vi "svpo_Average Array (real).vi"(6 "averages completed in":dbl, 7 "restart averaging":bool, 8 "exponential weight (10 %)":dbl=10.0 min=0.0 max=100.0 step=5.0, 9 "weighting mode":enum16{"Linear", "Exponential"}(ring), 10 "array":dbl[](array[numeric]) format="%.2p", 11 "previous average array":dbl[](array[numeric]) format="%.2p") -> (2 "averages completed out":dbl, 3 "average array":dbl[](array[numeric]) format="%.2p")   [LabVIEW 2017]
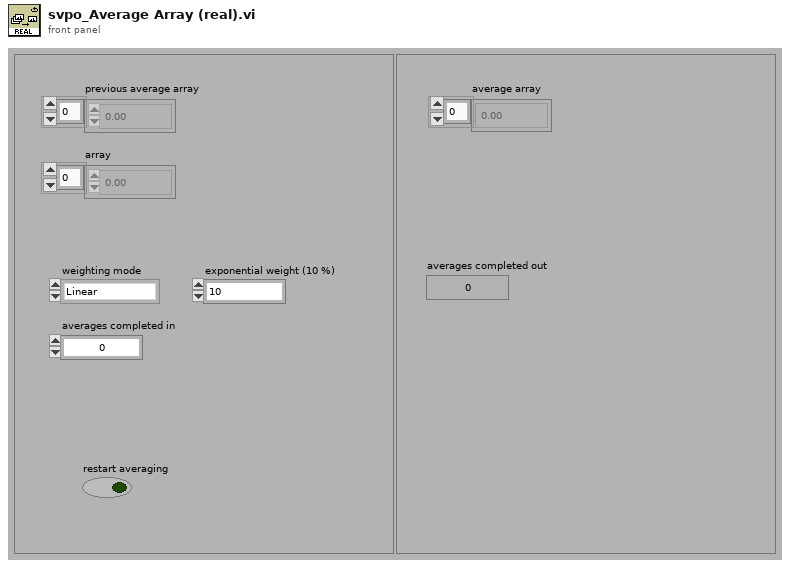
[diagram p1: front panel]
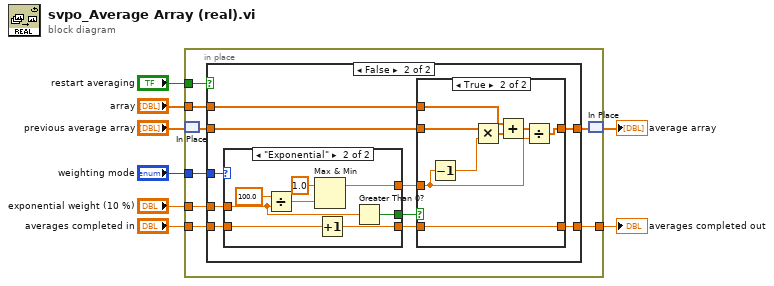
[diagram p0: block diagram]
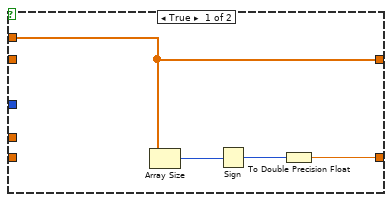
[diagram p2: hidden frame]
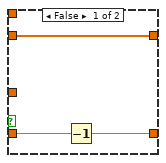
[diagram p3: hidden frame]
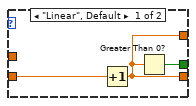
[diagram p4: hidden frame]
diagram:
  n1 = in-place {
    in-place-border: "weighting mode" -> [w16]
    in-place-border: "averages completed in" -> [w15]
    in-place-border: [w14] -> w6
    in-place-border: "array" -> [w13]
    in-place-border: "restart averaging" -> [w12]
    in-place-border: "exponential weight (10 %)" -> [w11]
    n2 = in-place-match #1("previous average array") -> (w10:dbl[])
    n3 = case shown="False" w12 {
      tunnel: [w19 w23] -> w14
      tunnel: w16 -> [_ w30]
      tunnel: w15 -> [_ w29]
      tunnel: w10 -> [_ w28]
      tunnel: w13 -> [w20 w27]
      tunnel: [w20 w26] -> w9
      tunnel: w11 -> [_ w25]
      frame True {
        n4 = Array Size(array=w20) -> (size(s)=w18:i32)
        n5 = Sign(1:w18) -> (0:w17:i32)
        n6 = To Double Precision Float(number=w17) -> (double precision float=w19:dbl)
      }
      frame False {
        n7 = case shown="\"Exponential\"" w30 {
          tunnel: w29 -> [w44 w51]
          tunnel: [w42 w52] -> w22
          tunnel: [w42 w48] -> w24
          tunnel: w25 -> [_ w46]
          tunnel: [w43 w45] -> w21
          frame "Linear", Default {
            n8 = Increment(x=w44) -> (x+1=w42:dbl)
            n9 = Greater Than 0?(x=w42) -> (x > 0?=w43:bool)
          }
          frame "Exponential" {
            n10 = Divide(x=100.0, y=w46) -> (x/y=w49:dbl)
            n11 = Max & Min(x=1.0 ("lower limit"), y=w49) -> (max(x,y)=w48:dbl)  [unwired: 1 out]
            n12 = Increment(x=w51) -> (x+1=w52:dbl)
            n13 = Greater Than 0?(x=w46) -> (x > 0?=w45:bool)
          }
        }
        n14 = case shown="True" w21 {
          tunnel: w28 -> [w33 w39]
          tunnel: w27 -> [_ w38]
          tunnel: [w33 w37] -> w26
          tunnel: w24 -> [_ w35]
          tunnel: [w31 w36] -> w23
          tunnel: w22 -> [w32 w36]
          frame False {
            n15 = Decrement(x=w32) -> (x-1=w31:dbl)
          }
          frame True {
            n16 = Decrement(x=w35) -> (x-1=w34:dbl)
            n17 = Multiply(x=w39, y=w34) -> (x*y=w40:dbl[])
            n18 = Add(x=w38, y=w40) -> (x+y=w41:dbl[])
            n19 = Divide(x=w41, y=w35) -> (x/y=w37:dbl[])
          }
        }
      }
    }
    n20 = in-place-match #1(w9) -> (→"average array":dbl[])
  }
  "averages completed out" <- w6
